vi "Inject Fan Controller.vi"(7 "Fan Controller Ref":refnum<data-value>, 8 "error in (no error)":errorcluster, 11 "iProcess Step Model in":refnum<class "iProcess Step Model.lvclass">) -> (0 "error out":errorcluster, 3 "iProcess Step Model out":refnum<class "iProcess Step Model.lvclass">)   [LabVIEW 2019, in "iProcess Step Model.lvclass"]
uses:
  <vilib>/gpm_packages/@cs/Car-wash/Source/iProcess Step Model/iProcess Step Model/iProcess Step Model.lvclass
  <vilib>/gpm_packages/@cs/Car-wash/Source/iFan Controller/iFan Controller.lvclass
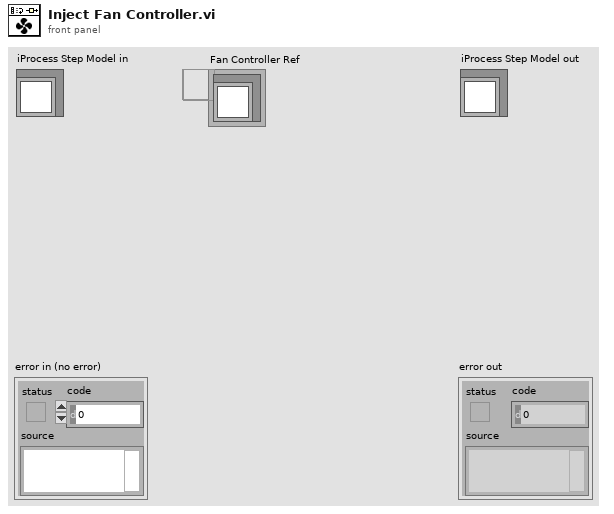
[diagram p1: front panel]
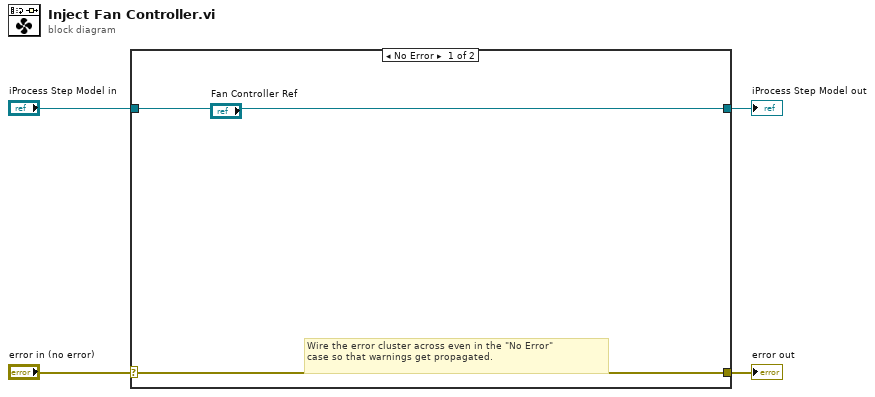
[diagram p0: block diagram]
diagram:
  n1 = case shown="No Error" "error in (no error)" {
    selector: "error in (no error)" -> [w5 w8]
    tunnel: [w5 w8] -> w3
    tunnel: [w6 w7] -> w1
    tunnel: "iProcess Step Model in" -> [w6 w7]
    frame No Error {
      # "Wire the error cluster across even in the \"No Error\"\ncase so that warnings get propagated."
    }
    frame Error {
    }
  }
  "error out" <- w3
  "iProcess Step Model out" <- w1
